vi "Get OCV SOC Curve.vi"(0 "reference in":refnum<class "Battery.lvclass">, 5 "Error In":errorcluster) -> (14 "reference out":refnum<class "Battery.lvclass">, 16 "OCV SOC Curve":dbl[][](array[numeric]), 19 "Error Out":errorcluster)   [LabVIEW 2023, in "Battery.lvclass"]
uses:
  Battery.lvclass
  Battery.lvclass/Battery.ctl
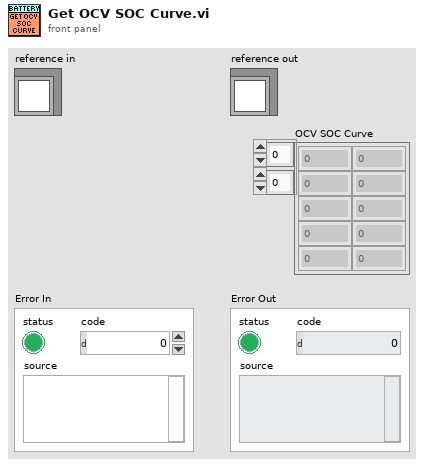
[diagram p1: front panel]
types:
  T1 = typedef "Battery.lvclass/ObjectAttributes.ctl" = cluster{"Python module":path, "Python Session":refnum<k35>, "PybammWrapper":refnum<k38>, "model loaded":bool, "simulation loaded":bool, "OCV SOC Curve":dbl[][]}
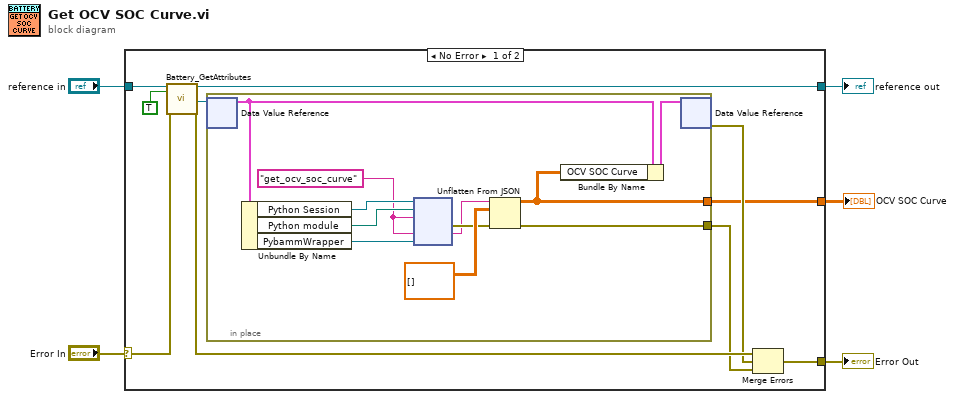
[diagram p0: block diagram]
diagram:
  n1 = case shown="No Error" "Error In" {
    selector: "Error In" -> [w14 w28]
    tunnel: [w12 w28] -> w4
    tunnel: [w13 w27] -> w2
    tunnel: "reference in" -> [w15 w27]
    tunnel: [w6 _] -> w1
    frame No Error {
      n2 = call "Battery_GetAttributes.vi"("reference in"=w15, "OnlyGetDvrReference(False)"=TRUE, "Error In"=w14) -> ("reference out"=w13:refnum<class "Battery.lvclass">, "DataRef"=w11:refnum<data-value>, "Error Out"=w9:errorcluster)  [unwired: 13 in, 1 out]
      n3 = in-place {
        in-place-border: [w17] -> w7
        in-place-border: [w16] -> w6
        w20 = "get_ocv_soc_curve" ("function name")
        n4 = in-place-dvr #1(w11) -> (w25:T1)  [unwired: 1 out]
        n5 = Unbundle By Name(w25) -> ("Python Session"=w23:refnum<k35>, "Python module"=w22:path, "PybammWrapper"=w24:refnum<k38>)
        n6 = node(w23, w22, w20, w20, w24) -> (w19:errorcluster, w18:string)  [unwired: 2 in, 3 out]
        n7 = Unflatten From JSON(JSON string=w18, type and defaults=dbl[][] [], error in (no error)=w19) -> (value=w16:dbl[][], error out=w17:errorcluster)  [unwired: 4 in]
        n8 = Bundle By Name(cluster=w25, "OCV SOC Curve"=w16) -> (w26:T1)
        n9 = in-place-dvr #1(w26) -> (w8:errorcluster)  [unwired: 1 out]
      }
      n10 = Merge Errors(w9, w8, w7) -> (w12:errorcluster)
    }
    frame Error {
    }
  }
  "Error Out" <- w4
  "reference out" <- w2
  "OCV SOC Curve" <- w1
